vi "RampInFlow.vi"(0 "object in":refnum<class "CetoniPump.lvclass">, 2 "Ramp In Settings":T1, 5 "error in (no error)":errorcluster) -> (14 "object out":refnum<class "CetoniPump.lvclass">, 16 "Target Level Reached":bool, 17 "Pump Status out":T2(array[cluster]), 19 "error out":errorcluster)   [LabVIEW 2021, in "CetoniPump.lvclass"]
uses:
  CetoniPump.lvclass
  CetoniPump.lvclass/CetoniPump.ctl
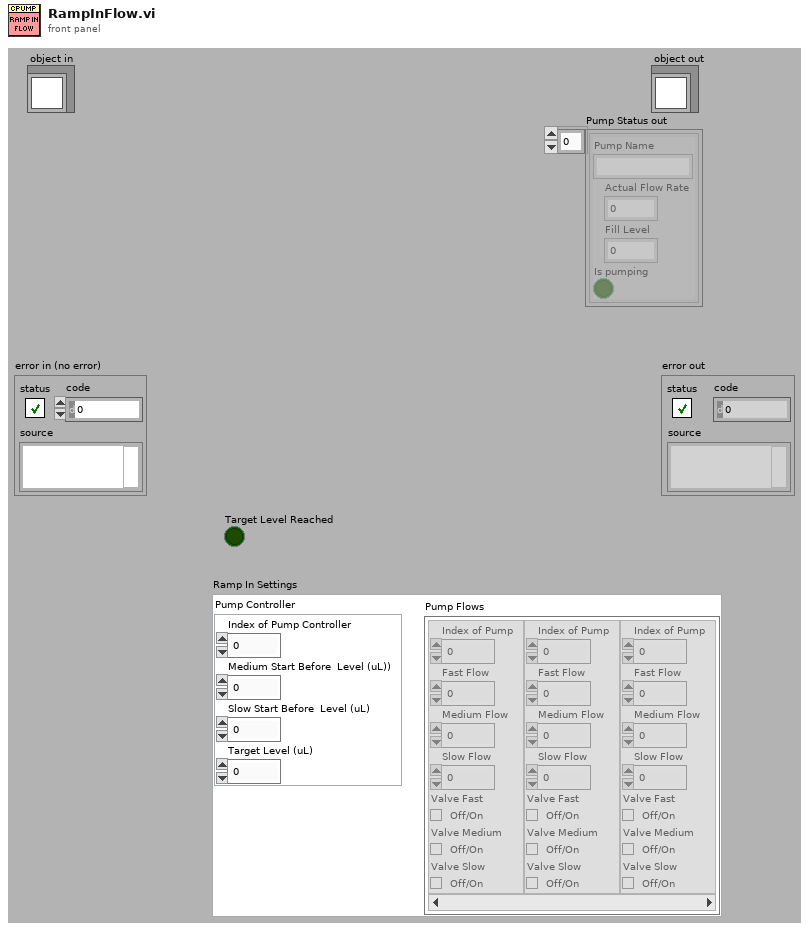
[diagram p1: front panel]
types:
  T1 = cluster{"Pump Controller":cluster{"Index of Pump Controller":u8, "Medium Start Before  Level (uL))":dbl, "Slow Start Before  Level (uL)":dbl, "Target Level (uL)":dbl}, "Pump Flows":cluster{"Index of Pump":u8, "Fast Flow":dbl, "Medium Flow":dbl, "Slow Flow":dbl, "Valve Fast":bool, "Valve Medium":bool, "Valve Slow":bool}[]}
  T2 = cluster{"Pump Name":string, "Actual Flow Rate":dbl, "Fill Level":dbl, "Is pumping":bool}[]
  T3 = cluster{"Index of Pump":u8, "Fast Flow":dbl, "Medium Flow":dbl, "Slow Flow":dbl, "Valve Fast":bool, "Valve Medium":bool, "Valve Slow":bool}[]
  T4 = cluster{"Pump Name":string, "Actual Flow Rate":dbl, "Fill Level":dbl, "Is pumping":bool}
  T5 = cluster{"Pump Handle":i64, "Pump Name":string, "Maximum Volume":dbl, "Maximum Flow Rate":dbl, "Flow Rate":dbl, "Target Level":dbl, "Valve Handle":i64, "Has Valve?":bool, "Actual valve position":i32}[]
  T6 = cluster{"Pump Handle":i64, "Pump Name":string, "Maximum Volume":dbl, "Maximum Flow Rate":dbl, "Flow Rate":dbl, "Target Level":dbl, "Valve Handle":i64, "Has Valve?":bool, "Actual valve position":i32}
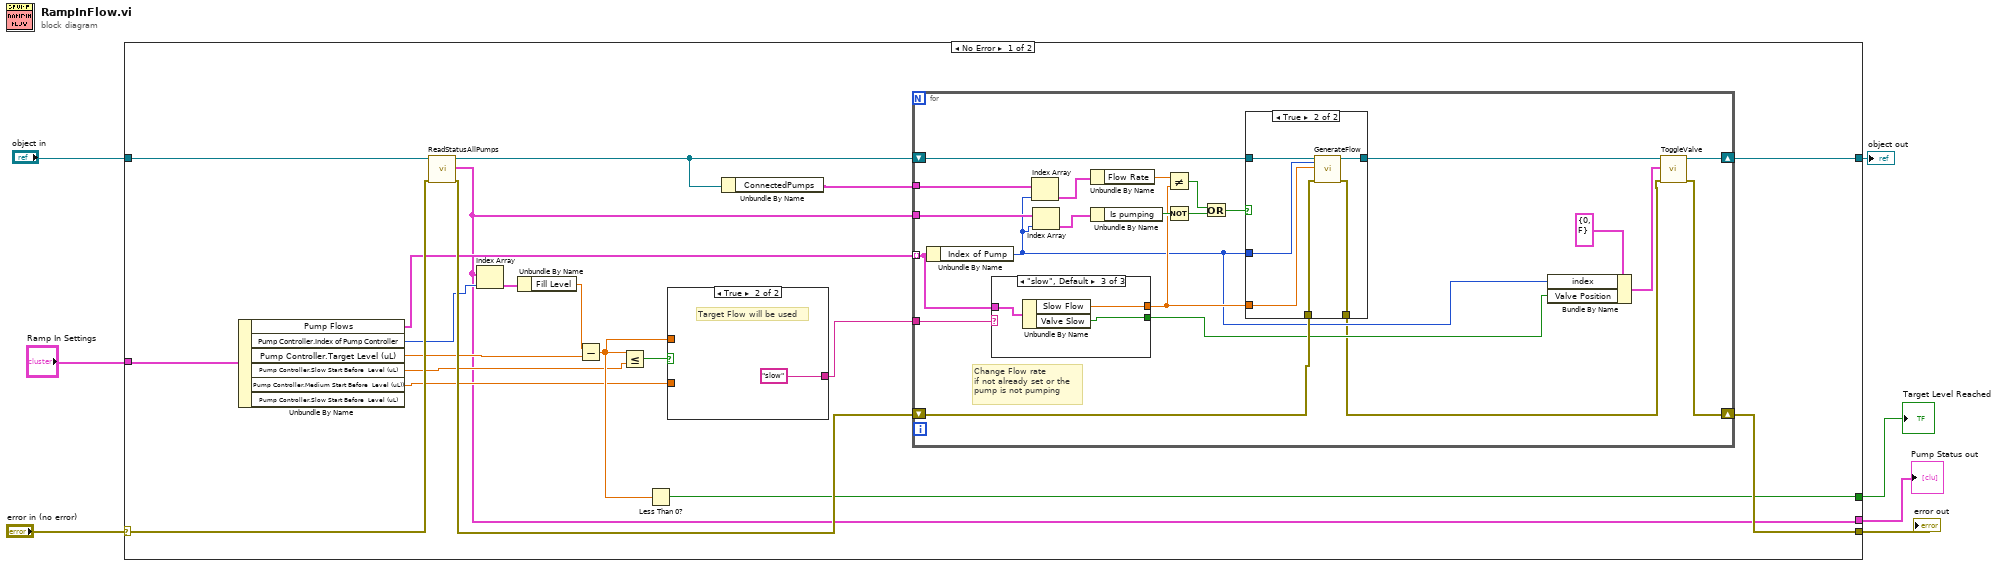
[diagram p0: block diagram]
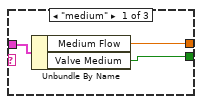
[diagram p2: hidden frame]
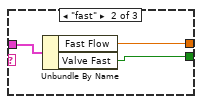
[diagram p3: hidden frame]
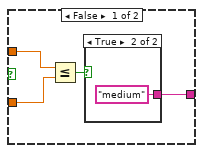
[diagram p5: hidden frame]
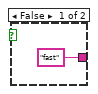
[diagram p6: hidden frame]
diagram:
  n1 = case shown="No Error" "error in (no error)" {
    selector: "error in (no error)" -> [w27 w75]
    tunnel: [w22 w75] -> w6
    tunnel: [w24 w74] -> w4
    tunnel: "object in" -> [w25 w74]
    tunnel: [w20 _] -> w3
    tunnel: [w9 _] -> w2
    tunnel: "Ramp In Settings" -> [w12 _]
    frame No Error {
      n2 = Unbundle By Name(w12) -> ("Pump Flows"=w11:T3, "Pump Controller.Index of Pump Controller"=w16:u8, "Pump Controller.Target Level (uL)"=w15:dbl, "Pump Controller.Slow Start Before  Level (uL)"=w14:dbl, "Pump Controller.Medium Start Before  Level (uL))"=w13:dbl)  [unwired: 1 out]
      n3 = call-dynamic "ReadStatusAllPumps.vi"("object in"=w25, "error in (no error)"=w27) -> ("object out"=w17:refnum<class "CetoniPump.lvclass">, "Array"=w9:T2, "error out"=w23:errorcluster)  [unwired: 15 in]
      n4 = Index Array(array=w9, index=w16) -> (element=w19:T4)
      n5 = Unbundle By Name(w19) -> ("Fill Level"=w18:dbl)
      n6 = Subtract(x=w18, y=w15) -> (x-y=w21:dbl)
      n7 = Less Or Equal?(x=w21, y=w14) -> (x <= y?=w26:bool)
      n8 = Less Than 0?(x=w21) -> (x < 0?=w20:bool)
      n9 = case shown="True" w26 {
        tunnel: w13 -> [w70 _]
        tunnel: w21 -> [w69 _]
        tunnel: [w67 "slow"] -> w8
        frame False {
          n10 = Less Or Equal?(x=w69, y=w70) -> (x <= y?=w68:bool)
          n11 = case shown="True" w68 {
            tunnel: ["fast" "medium"] -> w67
            frame False {
            }
            frame True {
            }
          }
        }
        frame True {
          # "Target Flow will be used"
        }
      }
      n12 = Unbundle By Name(w17) -> ("ConnectedPumps"=w10:T5)
      n13 = for {
        shift-right: [w30] -> w24
        shift-left: w17 -> [w48]
        shift-right: [w28] -> w22
        shift-left: w23 -> [w47]
        tunnel: w11 -> [w39] mode=indexing
        tunnel: w10 -> [w44]
        tunnel: w9 -> [w37]
        tunnel: w8 -> [w40]
        # "Change Flow rate \nif not already set or the \npump is not pumping"
        n14 = Unbundle By Name(w39) -> ("Index of Pump"=w33:u8)
        n15 = case shown="\"slow\", Default" w40 {
          tunnel: w39 -> [w52 w55 w58]
          tunnel: [w51 w54 w57] -> w38
          tunnel: [w50 w53 w56] -> w32
          frame "medium" {
            n16 = Unbundle By Name(w52) -> ("Medium Flow"=w51:dbl, "Valve Medium"=w50:bool)
          }
          frame "fast" {
            n17 = Unbundle By Name(w55) -> ("Fast Flow"=w54:dbl, "Valve Fast"=w53:bool)
          }
          frame "slow", Default {
            n18 = Unbundle By Name(w58) -> ("Slow Flow"=w57:dbl, "Valve Slow"=w56:bool)
          }
        }
        n19 = Index Array(array=w44, index=w33) -> (element=w43:T6)
        n20 = Index Array(array=w37, index=w33) -> (element=w36:T4)
        n21 = Unbundle By Name(w43) -> ("Flow Rate"=w49:dbl)
        n22 = Unbundle By Name(w36) -> ("Is pumping"=w46:bool)
        n23 = Not Equal?(x=w49, y=w38) -> (x != y?=w42:bool)
        n24 = Not(x=w46) -> (.not. x?=w41:bool)
        n25 = Or(x=w42, y=w41) -> (x .or. y?=w45:bool)
        n26 = case shown="True" w45 {
          tunnel: w48 -> [w60 w66]
          tunnel: [w60 w62] -> w31
          tunnel: w47 -> [w59 w65]
          tunnel: [w59 w64] -> w29
          tunnel: w33 -> [_ w61]
          tunnel: w38 -> [_ w63]
          frame False {
          }
          frame True {
            n27 = call-dynamic "GenerateFlow.vi"("object in"=w66, "index"=w61, "Flow Rate"=w63, "error in (no error)"=w65) -> ("object out"=w62:refnum<class "CetoniPump.lvclass">, "error out"=w64:errorcluster)  [unwired: 14 in]
          }
        }
        n28 = Bundle By Name(cluster=cluster{"index":i32, "Valve Position":bool} {"index"=0, "Valve Position"=FALSE} ("ValveControl"), "index"=w33, "Valve Position"=w32) -> (w35:cluster{"index":i32, "Valve Position":bool})
        n29 = call-dynamic "ToggleValve.vi"("object in"=w31, "ValveControl"=w35, "error in (no error)"=w29) -> ("object out"=w30:refnum<class "CetoniPump.lvclass">, "error out"=w28:errorcluster)  [unwired: 15 in]
      }
    }
    frame Error {
    }
  }
  "error out" <- w6
  "object out" <- w4
  "Target Level Reached" <- w3
  "Pump Status out" <- w2
